vi "Aula 10 19_10 Strings.vi"() -> ()   [LabVIEW 2020]
panel:
  out "Resultado num":string
  in  "Precisão":i16
  in  "Width":i16
  in  "Boolean":bool
  in  "Num":dbl
  in  "Ignore? (f)":bool
  in  "Replace all? (f)":bool
  out "Dps offset":i32
  out "Num subst":i32
  in  "Replace":string
  in  "Offset 3":i32
  out "Result 2":string
  in  "Search":string
  in  "String 3":string
  out "Replaced substring":string
  out "Result":string
  in  "Length":i32
  in  "Offset 2":i32
  in  "Substring 2":string
  in  "String 2":string
  out "Substring":string
  in  "Length":i32
  in  "Offset":i32
  in  "String":string
  out "string":string
  in  "Nome Completo 2":string
  out "Numeric":i32
  in  "Nome Completo":string
  in  "Stop Button":bool
  # "Offset determina onde começa (no 1 pula a primeira letra, no 2 a segunda e assim vai)"
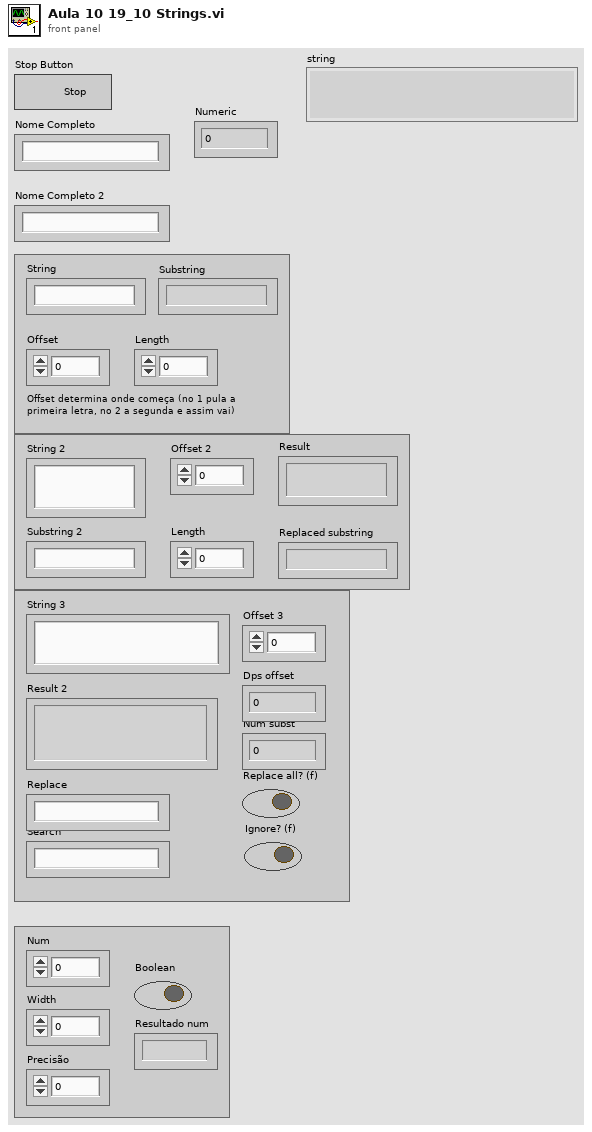
[diagram p1: front panel]
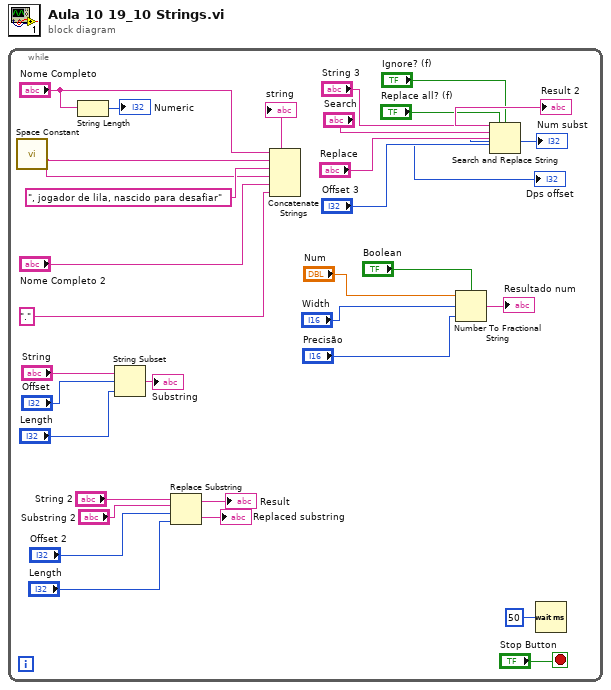
[diagram p0: block diagram]
diagram:
  n1 = while {
    stop <- "Stop Button" stop-if-true
    n2 = call <vilib>:"Space Constant.vi"() -> ("String"=w27:string)
    n3 = String Length(string="Nome Completo") -> (length=→"Numeric":i32)
    n4 = String Subset(string="String", offset (0)="Offset", length (rest)="Length") -> (substring=→"Substring":string)
    n5 = Replace Substring(2:"Length", 3:"Offset 2", 4:"Substring 2", 5:"String 2") -> (0:→"Replaced substring":string, 1:→"Result":string)
    n6 = Concatenate Strings("Nome Completo", w27, ", jogador de lila, nascido para desafiar" ("string"), w27, "Nome Completo 2", "." ("concatenated string")) -> (→"string":string)
    n7 = Number To Fractional String(use system decimal point (T)="Boolean", number="Num", width (-)="Width", precision (6)="Precisão") -> (F-format string=→"Resultado num":string)
    n8 = Search and Replace String(replace all?="Replace all? (f)", case sensitive?="Ignore? (f)", input string="String 3", search string="Search", replace string="Replace", offset="Offset 3") -> (result string=→"Result 2":string, number of replacements=→"Num subst":i32, offset past replacement=→"Dps offset":i32)  [unwired: 2 in, 1 out]
    n9 = Wait (ms)(milliseconds to wait=u32 50 ("millisecond timer value")) -> ()  [unwired: 1 out]
  }
